vi "Bluetooth - test.vi"() -> ()   [LabVIEW 2012]
panel:
  out "data out":string
  out "Device Name":string
  in  "time limit ms (10000)":i32
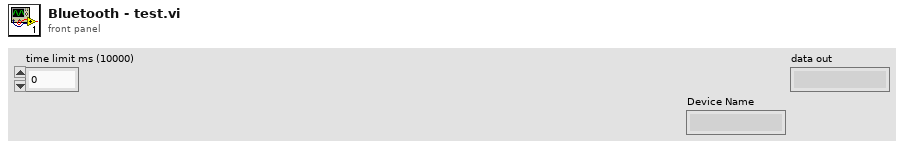
[diagram p1: front panel]
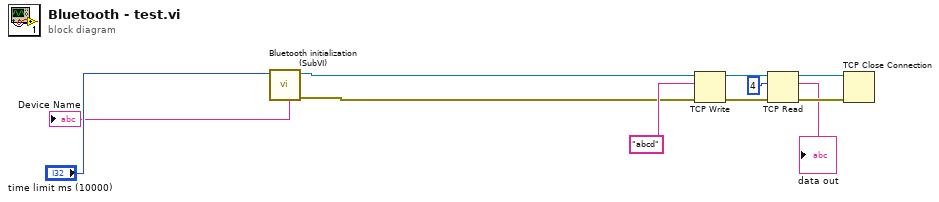
[diagram p0: block diagram]
diagram:
  n1 = call "Bluetooth initialization (SubVI).vi"("time limit ms (10000)"="time limit ms (10000)") -> ("error out"=w3:errorcluster, "Bluetooth Network Connection out"=w2:refnum<k31>, "Device Name"=→"Device Name":string)  [unwired: 5 in, 3 out]
  n2 = TCP Write(connection ID=w2, data in="abcd", error in (no error)=w3) -> (connection ID out=w8:refnum<k31>, error out=w9:errorcluster)  [unwired: 1 in, 1 out]
  n3 = TCP Read(connection ID=w8, bytes to read=4, error in (no error)=w9) -> (connection ID out=w6:refnum<k31>, data out=→"data out":string, error out=w5:errorcluster)  [unwired: 2 in]
  n4 = TCP Close Connection(connection ID=w6, error in (no error)=w5) -> ()  [unwired: 1 in, 2 out]
